vi "20210319_Shift_00_ATA_FPGA.vi"(6 "Scale":T5={"Scale_Step4"=1.0, "Scale_Step5"=1.0, "Scale_Step6"=1.0, "Scale_Step7"=1.0}, 7 "Input valid":bool, 8 "Index":u32, 9 "Enable":T1, 10 "frequency shift":fxp<+/-,48,0> format="%#.48g", 11 "Data in":fxp<+/-,18,1>) -> (1 "Q Shift Output":T3, 2 "I Shift Output":T3)   [LabVIEW 2018]
uses:
  FPGA_Controls/FPGA_Scale_Clust.ctl
  FPGA_Controls/FPGA_Probe_Clust.ctl
  FPGA_Controls/FPGA_ShiftOutput.ctl
  FPGA_Controls/FPGA_Shift_Enable.ctl
  FPGA_Controls/FPGA_Enable_Clust.ctl
  <instrlib>/_niInstr/DSP/v1/Shared/Public/IQ Data.ctl
  <instrlib>/_niInstr/DSP/v1/FPGA/Public/Sub VIs/Frequency Shift/Frequency Shift - 1 spc.vi
  <instrlib>/_niInstr/DSP/v1/Shared/niInstr DSP v1 Shared.lvlib
  <instrlib>/_niInstr/DSP/v1/FPGA/niInstr DSP v1 FPGA.lvlib
panel:
  out "Q Index":u32
  out "I Index":u32
  out "Q Probe":T4
  out "Q Data out":fxp<+/-,24,1>
  out "output valid":bool
  out "I Data out":fxp<+/-,24,1>
  out "I Probe":T4
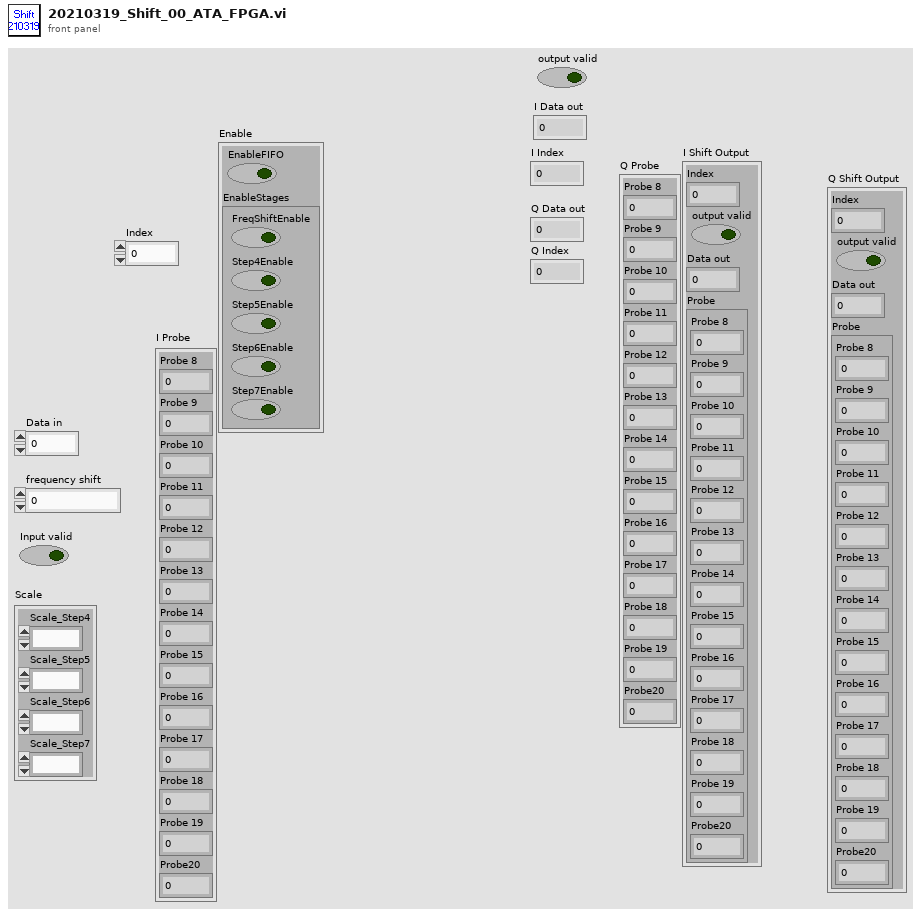
[diagram p1: front panel]
types:
  T1 = typedef "FPGA_Shift_Enable.ctl" = cluster{"EnableFIFO":bool, "EnableStages":T2}
  T2 = typedef "FPGA_Enable_Clust.ctl" = cluster{"FreqShiftEnable":bool, "Step4Enable":bool, "Step5Enable":bool, "Step6Enable":bool, "Step7Enable":bool}
  T3 = typedef "FPGA_ShiftOutput.ctl" = cluster{"Index":fxp<+/-,24,1>, "output valid":bool, "Data out":fxp<+/-,24,1>, "Probe":T4}
  T4 = typedef "FPGA_Probe_Clust.ctl" = cluster{"Probe 8":fxp<+/-,18,1>, "Probe 9":fxp<+/-,24,1>, "Probe 10":fxp<+/-,24,1>, "Probe 11":fxp<+/-,24,1>, "Probe 12":fxp<+/-,47,24>, "Probe 13":fxp<+/-,24,1>, "Probe 14":fxp<+/-,25,2>, "Probe 15":fxp<+/-,48,25>, "Probe 16":fxp<+/-,24,1>, "Probe 17":fxp<+/-,25,2>, "Probe 18":fxp<+/-,48,25>, "Probe 19":fxp<+/-,24,1>, "Probe20":fxp<+/-,24,1>}
  T5 = typedef "FPGA_Scale_Clust.ctl" = cluster{"Scale_Step4":fxp<+/-,23,23>, "Scale_Step5":fxp<+/-,23,23>, "Scale_Step6":fxp<+/-,23,23>, "Scale_Step7":fxp<+/-,23,23>}
  T6 = typedef "niInstr DSP v1 Shared.lvlib/IQ Data.ctl" = cluster{"I":fxp<+/-,18,1>, "Q":fxp<+/-,18,1>, "overflow":bool}
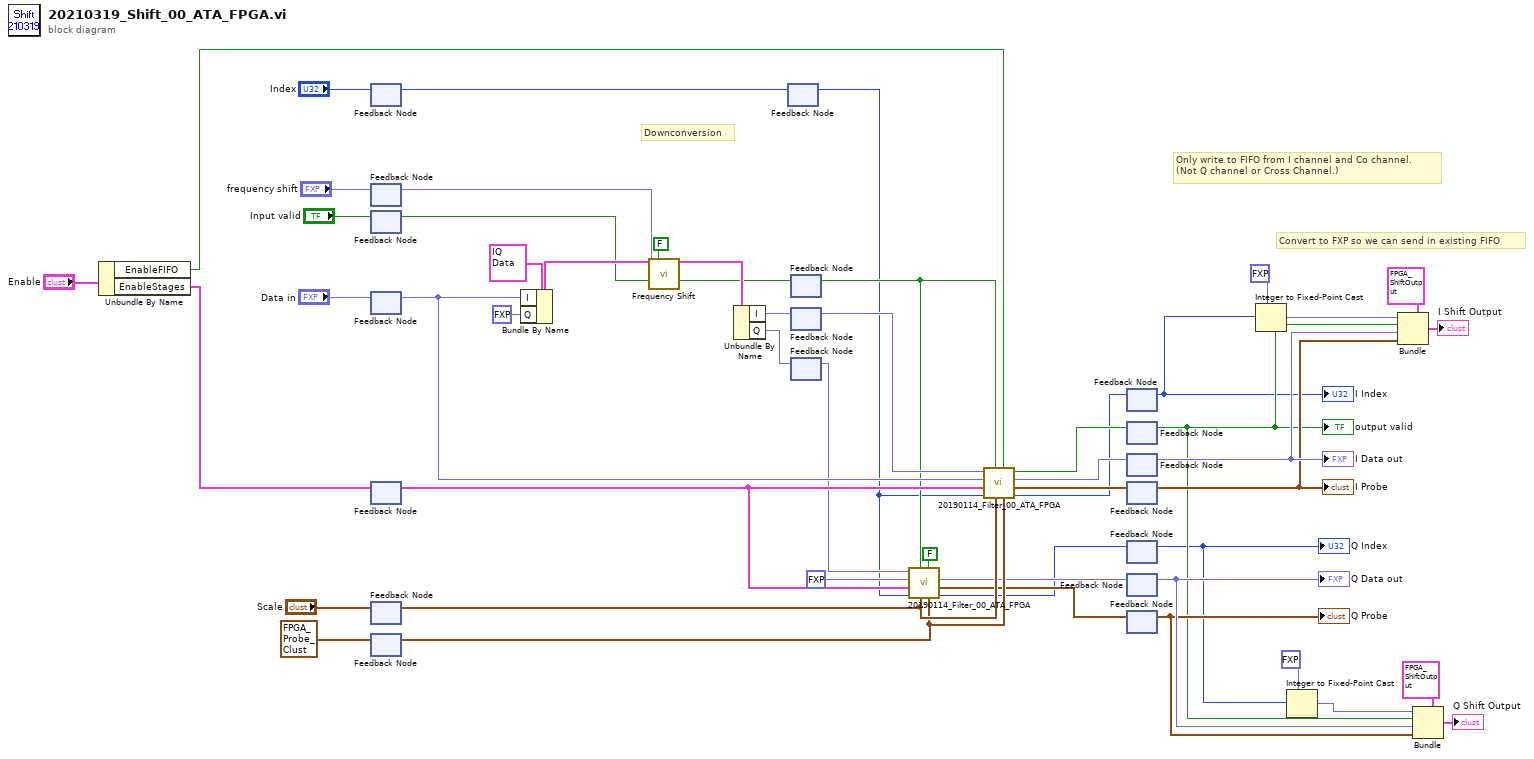
[diagram p0: block diagram]
diagram:
  # "Convert to FXP so we can send in existing FIFO"
  # "Only write to FIFO from I channel and Co channel.\n(Not Q channel or Cross Channel.)"
  # "Downconversion"
  n1 = Unbundle By Name("Enable") -> ("EnableFIFO"=w9:bool, "EnableStages"=w8:T2)
  n2 = feedback #1() -> (w22:u32)  [unwired: 1 in]
  n3 = feedback-in #1("Index") -> ()
  n4 = feedback #2() -> (w39:fxp<+/-,48,0>)  [unwired: 1 in]
  n5 = feedback-in #2("frequency shift") -> ()
  n6 = feedback #3() -> (w41:bool)  [unwired: 1 in]
  n7 = feedback-in #3("Input valid") -> ()
  n8 = feedback #4() -> (w44:fxp<+/-,18,1>)  [unwired: 1 in]
  n9 = feedback-in #4("Data in") -> ()
  n10 = feedback #5() -> (w43:T2)  [unwired: 1 in]
  n11 = feedback-in #5(w8) -> ()
  n12 = feedback #6() -> (w37:T5)  [unwired: 1 in]
  n13 = feedback-in #6("Scale") -> ()
  n14 = feedback #7() -> (w35:T4)  [unwired: 1 in]
  n15 = feedback-in #7(T4 {"Probe 8"=0.0, "Probe 9"=0.0, "Probe 10"=0.0, "Probe 11"=0.0, "Probe 12"=0.0, "Probe 13"=0.0, "Probe 14"=0.0, "Probe 15"=0.0, "Probe 16"=0.0, "Probe 17"=0.0, "Probe 18"=0.0, "Probe 19"=0.0, "Probe20"=0.0} ("Probe 9")) -> ()
  n16 = Bundle By Name(cluster=T6 {"I"=0.0, "Q"=0.0, "overflow"=FALSE} ("data"), "I"=w44, "Q"=fxp<+/-,18,1> 0.0) -> (w49:T6)
  n17 = call-poly <instrlib>:"Frequency Shift.vi"("data in"=w49, "reset"=FALSE, "frequency shift"=w39, "input valid"=w41) -> ("data out"=w48:T6, "output valid"=w31:bool)  [unwired: 8 in, 2 out]
  n18 = Unbundle By Name(w48) -> ("I"=w33:fxp<+/-,18,1>, "Q"=w34:fxp<+/-,18,1>)
  n19 = feedback #8() -> (w1:u32)  [unwired: 1 in]
  n20 = feedback-in #8(w22) -> ()
  n21 = feedback #9() -> (w30:bool)  [unwired: 1 in]
  n22 = feedback-in #9(w31) -> ()
  n23 = feedback #10() -> (w32:fxp<+/-,18,1>)  [unwired: 1 in]
  n24 = feedback-in #10(w33) -> ()
  n25 = feedback #11() -> ()  [unwired: 2 in]
  n26 = feedback-in #11(w34) -> ()
  n27 = call "20190114_Filter_00_ATA_FPGA.vi"("Probe 10"=w35, "EnableFIFO"=FALSE, "Scale"=w37, "output valid in"=w30, "Index"=w1, "Enable"=w43, "UnshiftedData"=fxp<+/-,18,1> 0.0, "ShiftedData"=w34) -> ("Index out"=w20:u32, "Probe 9"=w25:T4, "fixed-point type"=w26:fxp<+/-,24,1>)  [unwired: 1 out]
  n28 = call "20190114_Filter_00_ATA_FPGA.vi"("Probe 10"=w35, "EnableFIFO"=w9, "Scale"=w37, "output valid in"=w30, "Index"=w1, "Enable"=w43, "UnshiftedData"=w44, "ShiftedData"=w32) -> ("Index out"=w21:u32, "Probe 9"=w27:T4, "fixed-point type"=w28:fxp<+/-,24,1>, "output valid out"=w29:bool)
  n29 = feedback #12() -> (w3:u32)  [unwired: 1 in]
  "I Index" <- w3
  n30 = feedback-in #12(w21) -> ()
  n31 = feedback #13() -> (w11:bool)  [unwired: 1 in]
  "output valid" <- w11
  n32 = feedback-in #13(w29) -> ()
  n33 = feedback #14() -> (w19:fxp<+/-,24,1>)  [unwired: 1 in]
  "I Data out" <- w19
  n34 = feedback-in #14(w28) -> ()
  n35 = feedback #15() -> (w18:T4)  [unwired: 1 in]
  "I Probe" <- w18
  n36 = feedback-in #15(w27) -> ()
  n37 = feedback #16() -> (w2:u32)  [unwired: 1 in]
  "Q Index" <- w2
  n38 = feedback-in #16(w20) -> ()
  n39 = feedback #17() -> (w13:fxp<+/-,24,1>)  [unwired: 1 in]
  "Q Data out" <- w13
  n40 = feedback-in #17(w26) -> ()
  n41 = feedback #18() -> (w12:T4)  [unwired: 1 in]
  "Q Probe" <- w12
  n42 = feedback-in #18(w25) -> ()
  n43 = Integer to Fixed-Point Cast(fixed-point type=fxp<+/-,24,1> 0.0, integer=w3) -> (fixed-point=w6:fxp<+/-,24,1>)
  n44 = Integer to Fixed-Point Cast(fixed-point type=fxp<+/-,24,1> 0.0, integer=w2) -> (fixed-point=w4:fxp<+/-,24,1>)
  n45 = Bundle(cluster=T3 {"Index"=0.0, "output valid"=FALSE, "Data out"=0.0, "Probe"={"Probe 8"=0.0, "Probe 9"=0.0, "Probe 10"=0.0, "Probe 11"=0.0, "Probe 12"=0.0, "Probe 13"=0.0, "Probe 14"=0.0, "Probe 15"=0.0, "Probe 16"=0.0, "Probe 17"=0.0, "Probe 18"=0.0, "Probe 19"=0.0, "Probe20"=0.0}} ("Shift Output"), "Index"=w6, "output valid"=w11, "Data out"=w19, "Probe"=w18) -> (→"I Shift Output":T3)
  n46 = Bundle(cluster=T3 {"Index"=0.0, "output valid"=FALSE, "Data out"=0.0, "Probe"={"Probe 8"=0.0, "Probe 9"=0.0, "Probe 10"=0.0, "Probe 11"=0.0, "Probe 12"=0.0, "Probe 13"=0.0, "Probe 14"=0.0, "Probe 15"=0.0, "Probe 16"=0.0, "Probe 17"=0.0, "Probe 18"=0.0, "Probe 19"=0.0, "Probe20"=0.0}} ("Shift Output"), "Index"=w4, "output valid"=w11, "Data out"=w13, "Probe"=w12) -> (→"Q Shift Output":T3)
